vi "OE1022D Example All Data.vi"() -> ()   [LabVIEW 2014]
panel:
  out "θh1 (°) 2":sgl caption="θh1 (deg)" format="%.2f"
  out "Rh1 2":sgl caption="Rh1 (Vrms)" format="%.3p"
  out "Yh1 2":sgl caption="Yh1 (Vrms)" format="%.3p"
  out "Xh1 2":sgl caption="Xh1 (Vrms)" format="%.3p"
  out "Xh2 2":sgl caption="Xh2 (Vrms)" format="%.3p"
  out "Yh2 2":sgl caption="Yh2 (Vrms)" format="%.3p"
  out "Rh2 2":sgl caption="Rh2 (Vrms)" format="%.3p"
  out "噪声 2":sgl caption="Noise(Vrms)" format="%.3p"
  out "频率 (Hz) 2":sgl caption="Freq (Hz)" format="%#.3f"
  out "θ (°) 2":sgl caption="θ (deg)" format="%.2f"
  out "R 2":sgl caption="R (Vrms)" format="%.3p"
  out "Y 2":sgl caption="Y (Vrms)" format="%.3p"
  out "θh2 (°) 2":sgl caption="θh2 (deg)" format="%.2f"
  out "X 2":sgl caption="X (Vrms)" format="%.3p"
  out "Yh1":sgl caption="Yh1 (Vrms)" format="%.3p"
  out "Xh1":sgl caption="Xh1 (Vrms)" format="%.3p"
  out "θh2 (°)":sgl caption="θh2 (deg)" format="%.2f"
  out "Yh2":sgl caption="Yh2 (Vrms)" format="%.3p"
  out "Xh2":sgl caption="Xh2 (Vrms)" format="%.3p"
  out "Rh2":sgl caption="Rh2 (Vrms)" format="%.3p"
  out "θh1 (°)":sgl caption="θh1 (deg)" format="%.2f"
  out "Rh1":sgl caption="Rh1 (Vrms)" format="%.3p"
  out "噪声":sgl caption="Noise(Vrms)" format="%.3p"
  out "频率 (Hz)":sgl caption="Freq (Hz)" format="%#.3f"
  out "θ (°)":sgl caption="θ (deg)" format="%.2f"
  out "Y":sgl caption="Y (Vrms)" format="%.3p"
  out "X":sgl caption="X (Vrms)" format="%.3p"
  out "R":sgl caption="R (Vrms)" format="%.3p"
  out "AUX-ADC2 (V)":sgl format="%.3f"
  out "AUX-ADC1 (V)":sgl format="%.3f"
  out "AUX-ADC3 (V)":sgl format="%.3f"
  out "AUX-ADC4 (V)":sgl format="%.3f"
  out "错误输出":errorcluster
  out "序列号":string
  in  "OE1022D":refnum<visa-resource-name>
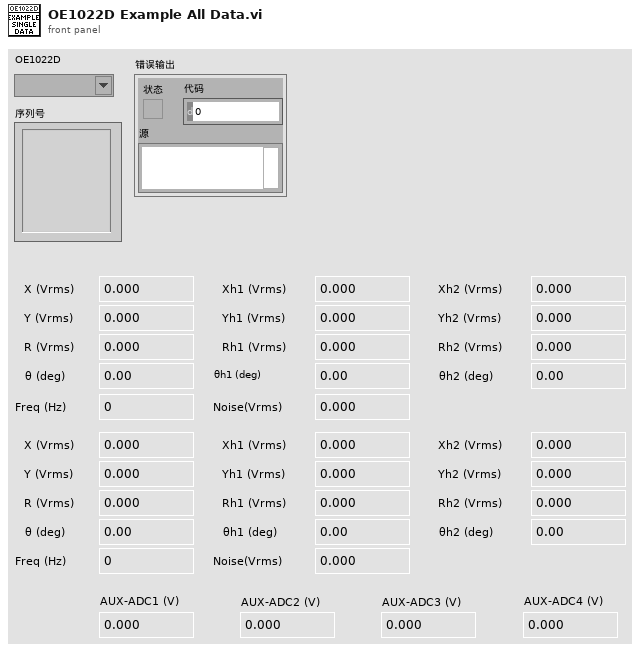
[diagram p1: front panel]
types:
  T1 = cluster{"AD1":dbl[], "AD2":dbl[], "AD3":dbl[], "AD4":dbl[]}
  T2 = cluster{"XB":dbl[], "YB":dbl[], "FrequencyB":dbl[], "NoiseB":dbl[], "Xh1B":dbl[], "Yh1B":dbl[], "Xh2B":dbl[], "Yh2B":dbl[], "Xh2B":dbl[]}
  T3 = cluster{"XA":dbl[], "YA":dbl[], "FrequencyA":dbl[], "NoiseA":dbl[], "Xh1A":dbl[], "Yh1A":dbl[], "Xh2A":dbl[], "Yh2A":dbl[]}
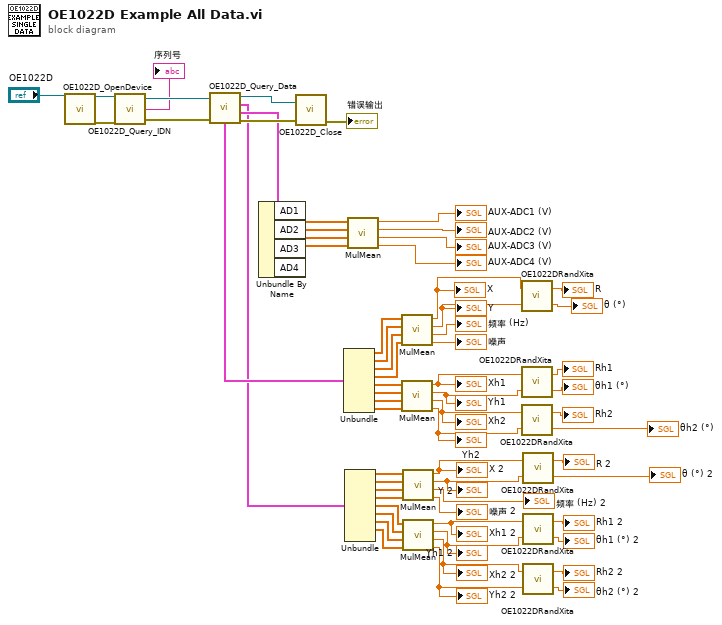
[diagram p0: block diagram]
diagram:
  n1 = call "OE1022D_OpenDevice.vi"("VISA resource name"="OE1022D") -> ("VISA资源名称输出"=w64:refnum<visa-resource-name>, "错误输出"=w61:errorcluster)  [unwired: 17 in]
  n2 = call "OE1022D_Query_IDN.vi"("错误输入（无错误）"=w61, "VISA resource name"=w64) -> ("错误输出"=w62:errorcluster, "序列号"=→"序列号":string, "VISA resource name out"=w57:refnum<visa-resource-name>)  [unwired: 1 in]
  n3 = call "OE1022D_Query_Data.vi"("错误输入（无错误）"=w62, "VISA resource name"=w57) -> ("error out"=w59:errorcluster, "输出簇ADC"=w2:T1, "输出簇B"=w1:T2, "VISA resource name out"=w60:refnum<visa-resource-name>, "输出簇A"=w3:T3)  [unwired: 3 in]
  n4 = Unbundle By Name(w2) -> ("AD1"=w52:dbl[], "AD2"=w53:dbl[], "AD3"=w54:dbl[], "AD4"=w55:dbl[])
  n5 = call "OE1022D_Close.vi"("错误输入（无错误）"=w59, "VISA resource name"=w60) -> ("错误输出"=→"错误输出":errorcluster)  [unwired: 1 in]
  n6 = Unbundle(w3) -> ("XA"=w8:dbl[], "YA"=w9:dbl[], "FrequencyA"=w10:dbl[], "NoiseA"=w11:dbl[], "Xh1A"=w18:dbl[], "Yh1A"=w19:dbl[], "Xh2A"=w20:dbl[], "Yh2A"=w21:dbl[])
  n7 = Unbundle(w1) -> ("XB"=w37:dbl[], "YB"=w36:dbl[], "FrequencyB"=w35:dbl[], "NoiseB"=w34:dbl[], "Xh1B"=w33:dbl[], "Yh1B"=w32:dbl[], "Xh2B"=w31:dbl[], "Yh2B"=w30:dbl[])  [unwired: 1 out]
  n8 = call "MulMean.vi"("IN 4"=w55, "IN 3"=w54, "IN 2"=w53, "IN 1"=w52) -> ("mean 4"=→"AUX-ADC4 (V)":dbl, "mean 3"=→"AUX-ADC3 (V)":dbl, "mean 2"=→"AUX-ADC2 (V)":dbl, "mean 1"=→"AUX-ADC1 (V)":dbl)  [unwired: 4 in]
  n9 = call "MulMean.vi"("IN 4"=w11, "IN 3"=w10, "IN 2"=w9, "IN 1"=w8) -> ("mean 4"=→"噪声":dbl, "mean 3"=→"频率 (Hz)":dbl, "mean 2"=w14:dbl, "mean 1"=w13:dbl)  [unwired: 4 in]
  "X" <- w13
  "Y" <- w14
  n10 = call "MulMean.vi"("IN 4"=w21, "IN 3"=w20, "IN 2"=w19, "IN 1"=w18) -> ("mean 4"=w27:dbl, "mean 3"=w26:dbl, "mean 2"=w23:dbl, "mean 1"=w22:dbl)  [unwired: 4 in]
  "Xh2" <- w26
  "Yh2" <- w27
  "Xh1" <- w22
  "Yh1" <- w23
  n11 = call "MulMean.vi"("IN 4"=w34, "IN 3"=w35, "IN 2"=w36, "IN 1"=w37) -> ("mean 4"=→"噪声 2":dbl, "mean 3"=→"频率 (Hz) 2":dbl, "mean 2"=w43:dbl, "mean 1"=w42:dbl)  [unwired: 4 in]
  "X 2" <- w42
  "Y 2" <- w43
  n12 = call "MulMean.vi"("IN 4"=w30, "IN 3"=w31, "IN 2"=w32, "IN 1"=w33) -> ("mean 4"=w49:dbl, "mean 3"=w48:dbl, "mean 2"=w45:dbl, "mean 1"=w44:dbl)  [unwired: 4 in]
  "Yh2 2" <- w49
  "Xh2 2" <- w48
  "Xh1 2" <- w44
  "Yh1 2" <- w45
  n13 = call "OE1022DRandXita.vi"("Y"=w14, "X"=w13) -> ("θ (°)"=→"θ (°)":dbl, "R"=→"R":dbl)
  n14 = call "OE1022DRandXita.vi"("Y"=w23, "X"=w22) -> ("θ (°)"=→"θh1 (°)":dbl, "R"=→"Rh1":dbl)
  n15 = call "OE1022DRandXita.vi"("Y"=w27, "X"=w26) -> ("θ (°)"=→"θh2 (°)":dbl, "R"=→"Rh2":dbl)
  n16 = call "OE1022DRandXita.vi"("Y"=w43, "X"=w42) -> ("θ (°)"=→"θ (°) 2":dbl, "R"=→"R 2":dbl)
  n17 = call "OE1022DRandXita.vi"("Y"=w45, "X"=w44) -> ("θ (°)"=→"θh1 (°) 2":dbl, "R"=→"Rh1 2":dbl)
  n18 = call "OE1022DRandXita.vi"("Y"=w49, "X"=w48) -> ("θ (°)"=→"θh2 (°) 2":dbl, "R"=→"Rh2 2":dbl)
